vi "lab2_subVI.vi"(6 "System Params":cluster{"b":dbl, "a0":dbl, "a1":dbl, "a2":dbl}, 8 "Velocity":dbl, 9 "Position":dbl, 10 "Input":dbl, 11 "dt":dbl) -> (2 "Position":dbl, 3 "Velocity":dbl)   [LabVIEW 2020]
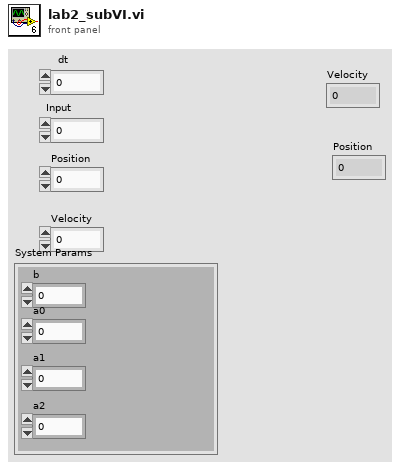
[diagram p1: front panel]
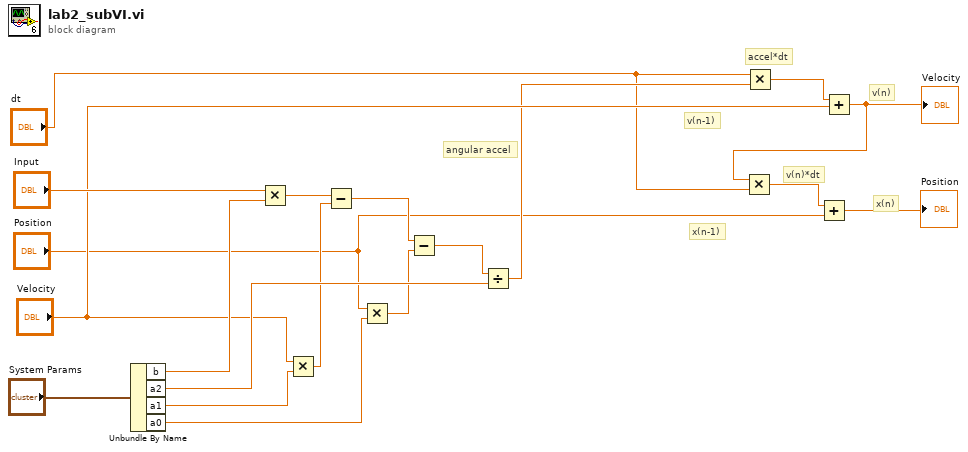
[diagram p0: block diagram]
diagram:
  # "x(n-1)"
  # "v(n-1)"
  # "x(n)"
  # "v(n)*dt"
  # "v(n)"
  # "angular accel"
  # "accel*dt"
  n1 = Unbundle By Name("System Params") -> ("b"=w18:dbl, "a2"=w16:dbl, "a1"=w15:dbl, "a0"=w14:dbl)
  n2 = Multiply(x="Input", y=w18) -> (x*y=w12:dbl)
  n3 = Multiply(x="Velocity", y=w15) -> (x*y=w13:dbl)
  n4 = Subtract(x=w12, y=w13) -> (x-y=w11:dbl)
  n5 = Multiply(x="Position", y=w14) -> (x*y=w10:dbl)
  n6 = Subtract(x=w11, y=w10) -> (x-y=w9:dbl)
  n7 = Divide(x=w9, y=w16) -> (x/y=w6:dbl)
  n8 = Multiply(x="dt", y=w6) -> (x*y=w8:dbl)
  n9 = Add(x=w8, y="Velocity") -> (x+y=w2:dbl)
  "Velocity" <- w2
  n10 = Multiply(x=w2, y="dt") -> (x*y=w5:dbl)
  n11 = Add(x=w5, y="Position") -> (x+y=→"Position":dbl)
